vi "Write Visa.vi"(8 "error in (no error)":errorcluster, 10 "write buffer":string, 11 "VisaComms in":refnum<class "VisaComms.lvclass">) -> (0 "error out":errorcluster, 2 "return count":u32, 3 "VisaComms out":refnum<class "VisaComms.lvclass">)   [LabVIEW 2020, in "CTI.lvlib" / "VisaComms.lvclass"]
uses:
  VisaComms.lvclass
  VisaComms.lvclass/VisaComms.ctl
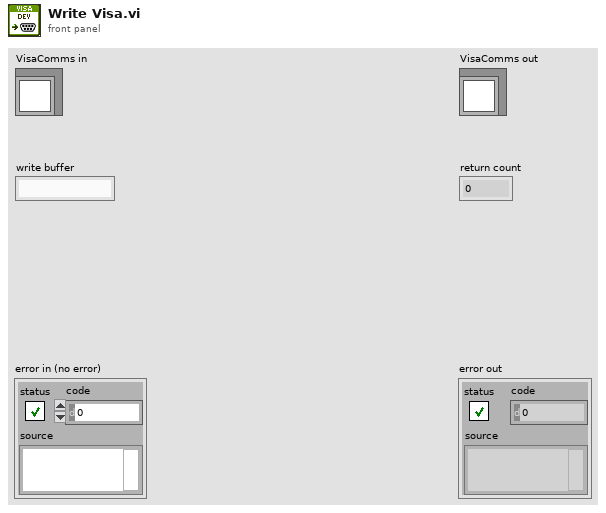
[diagram p1: front panel]
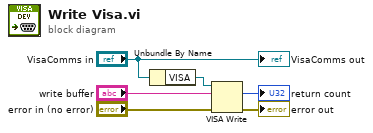
[diagram p0: block diagram]
diagram:
  n1 = Unbundle By Name("VisaComms in") -> ("VISA"=w6:refnum<visa-resource-name>)
  n2 = VISA Write(VISA resource name=w6, write buffer="write buffer", error in (no error)="error in (no error)") -> (return count=→"return count":u32, error out=→"error out":errorcluster)  [unwired: 1 out]
  "VisaComms out" <- "VisaComms in"
